vi "Finish Stream.vi"(8 "error in (no error)":errorcluster, 11 "Andor Camera in":refnum<class "Andor Camera.lvclass">) -> (0 "error out":errorcluster, 3 "Andor Camera out":refnum<class "Andor Camera.lvclass">)   [LabVIEW 2018, in "Andor Camera.lvlib" / "Andor Camera.lvclass"]
uses:
  Andor Camera.lvclass
  Camera/Camera.lvclass
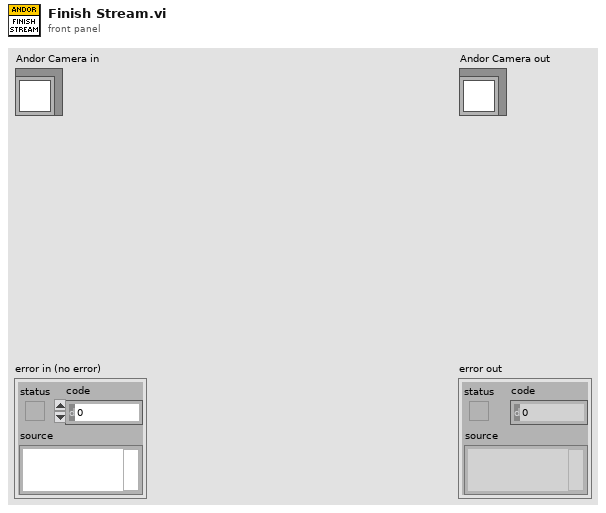
[diagram p1: front panel]
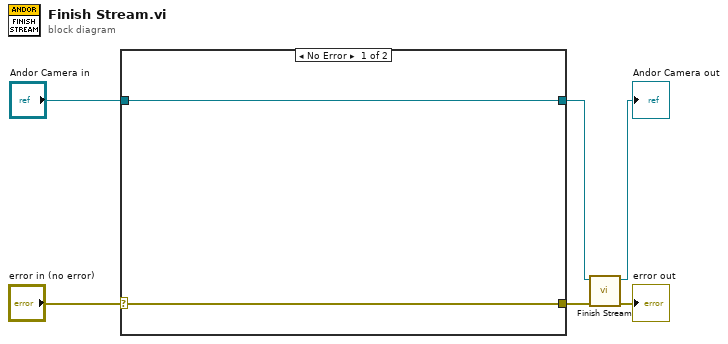
[diagram p0: block diagram]
diagram:
  n1 = case shown="No Error" "error in (no error)" {
    selector: "error in (no error)" -> [w7 w9]
    tunnel: [w7 w9] -> w3
    tunnel: "Andor Camera in" -> [w8 w10]
    tunnel: [w8 w10] -> w1
    frame No Error {
    }
    frame Error {
    }
  }
  n2 = call-parent "Finish Stream.vi"("error in (no error)"=w3, "Camera in"=w1) -> ("error out"=→"error out":errorcluster, "Camera out"=→"Andor Camera out":refnum<class "Andor Camera.lvclass">)  [unwired: 8 in]
